vi "Get All Data from registers list.vi"(8 "error in (no error)":errorcluster, 11 "Sensor General Class in":refnum<class "Sensor General Class.lvclass">) -> (0 "error out":errorcluster, 2 "Data":sgl[](array[numeric]), 3 "Sensor General Class out":refnum<class "Sensor General Class.lvclass">)   [LabVIEW 2020, in "Sensor General Class.lvclass"]
uses:
  Sensor General Class.lvclass
  Sensor General Class.lvclass/Sensor General Class.ctl
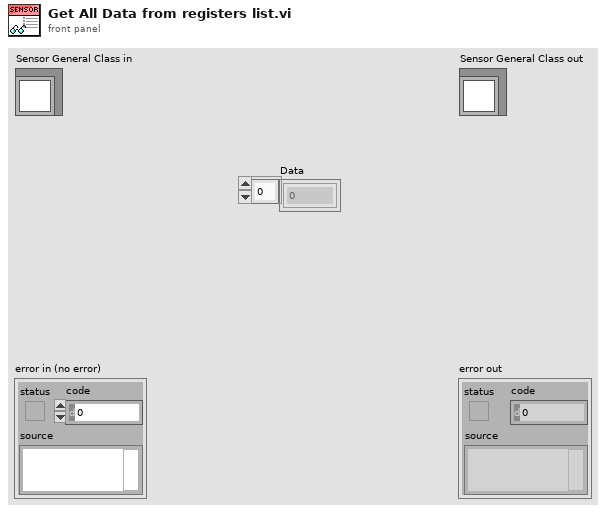
[diagram p1: front panel]
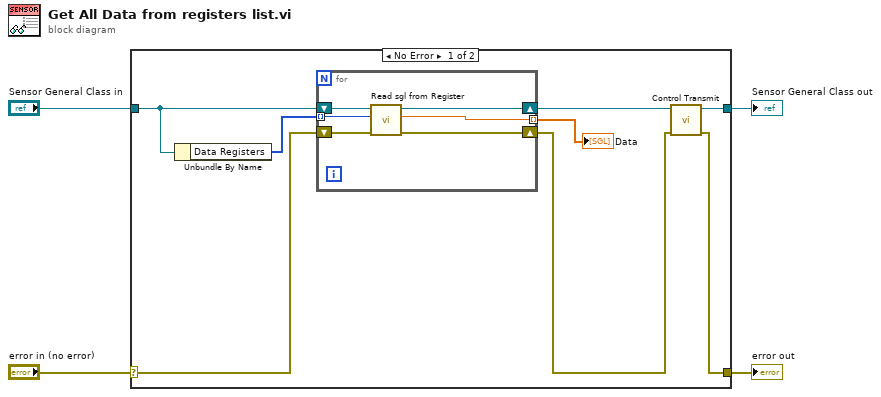
[diagram p0: block diagram]
diagram:
  n1 = case shown="No Error" "error in (no error)" {
    selector: "error in (no error)" -> [w10 w20]
    tunnel: [w5 w20] -> w3
    tunnel: [w7 w19] -> w1
    tunnel: "Sensor General Class in" -> [w12 w19]
    frame No Error {
      n2 = Unbundle By Name(w12) -> ("Data Registers"=w11:u16[])
      n3 = for {
        tunnel: w11 -> [w17] mode=indexing
        shift-right: [w16] -> w6
        shift-left: w10 -> [w13]
        shift-right: [w15] -> w8
        shift-left: w12 -> [w18]
        tunnel: [w14] -> w9 mode=indexing
        n4 = call-dynamic "Read sgl from Register.vi"("error in (no error)"=w13, "Start Register"=w17, "Sensor General Class in"=w18) -> ("error out"=w16:errorcluster, "Data"=w14:sgl, "Sensor General Class out"=w15:refnum<class "Sensor General Class.lvclass">)  [unwired: 6 in]
      }
      "Data" <- w9
      n5 = call-dynamic "Control Transmit.vi"("error in (no error)"=w6, "Sensor General Class in"=w8) -> ("error out"=w5:errorcluster, "Sensor General Class out"=w7:refnum<class "Sensor General Class.lvclass">)  [unwired: 8 in]
    }
    frame Error {
    }
  }
  "error out" <- w3
  "Sensor General Class out" <- w1
